vi "Movement Test (Remote Control).vi"() -> ()   [LabVIEW 2019]
uses:
  SubVIs/Move Type.ctl
  LINX-PCA9865 PWM/LINX-PCA9865 PWM.lvclass
  LINX-PCA9865 PWM/LINX-PCA9865 PWM.lvclass/LINX-PCA9865 PWM.ctl
  LINX-PCA9865 PWM/Write LINX Resource.vi
  LINX-PCA9865 PWM/Write I2C Slave Address (0x40).vi
  LINX-PCA9865 PWM/Write LINX I2C Channel.vi
  LINX-PCA9865 PWM/Read LINX Resource.vi
  <vilib>/MakerHub/LINX/Public/Utilities/Open Local.vi
  <vilib>/MediaMongrels Ltd/Message Queue Helper/MessageQueueHelper.lvlib
  <vilib>/MakerHub/LINX/LMH-LINX.lvlib
panel:
  in  "Array":T1[](array[typedef])=[{"Option"="Forward", "Left"=27.0, "Right"=10.0, "Duration"=3.0}, {"Option"="Back", "Left"=-14.0, "Right"=-28.0, "Duration"=3.0}, {"Option"="Left", "Left"=-10.0, "Right"=6.0, "Duration"=0.5}, {"Option"="Right", "Left"=25.0, "Right"=-25.0, "Duration"=0.5}]
  in  "Exit":bool
  in  "Stop":bool
  in  "Left":bool
  in  "Right":bool
  in  "Back":bool
  in  "Forward":bool
  out "Frequency (Hz)":dbl
  out "Drives Enabled?":bool
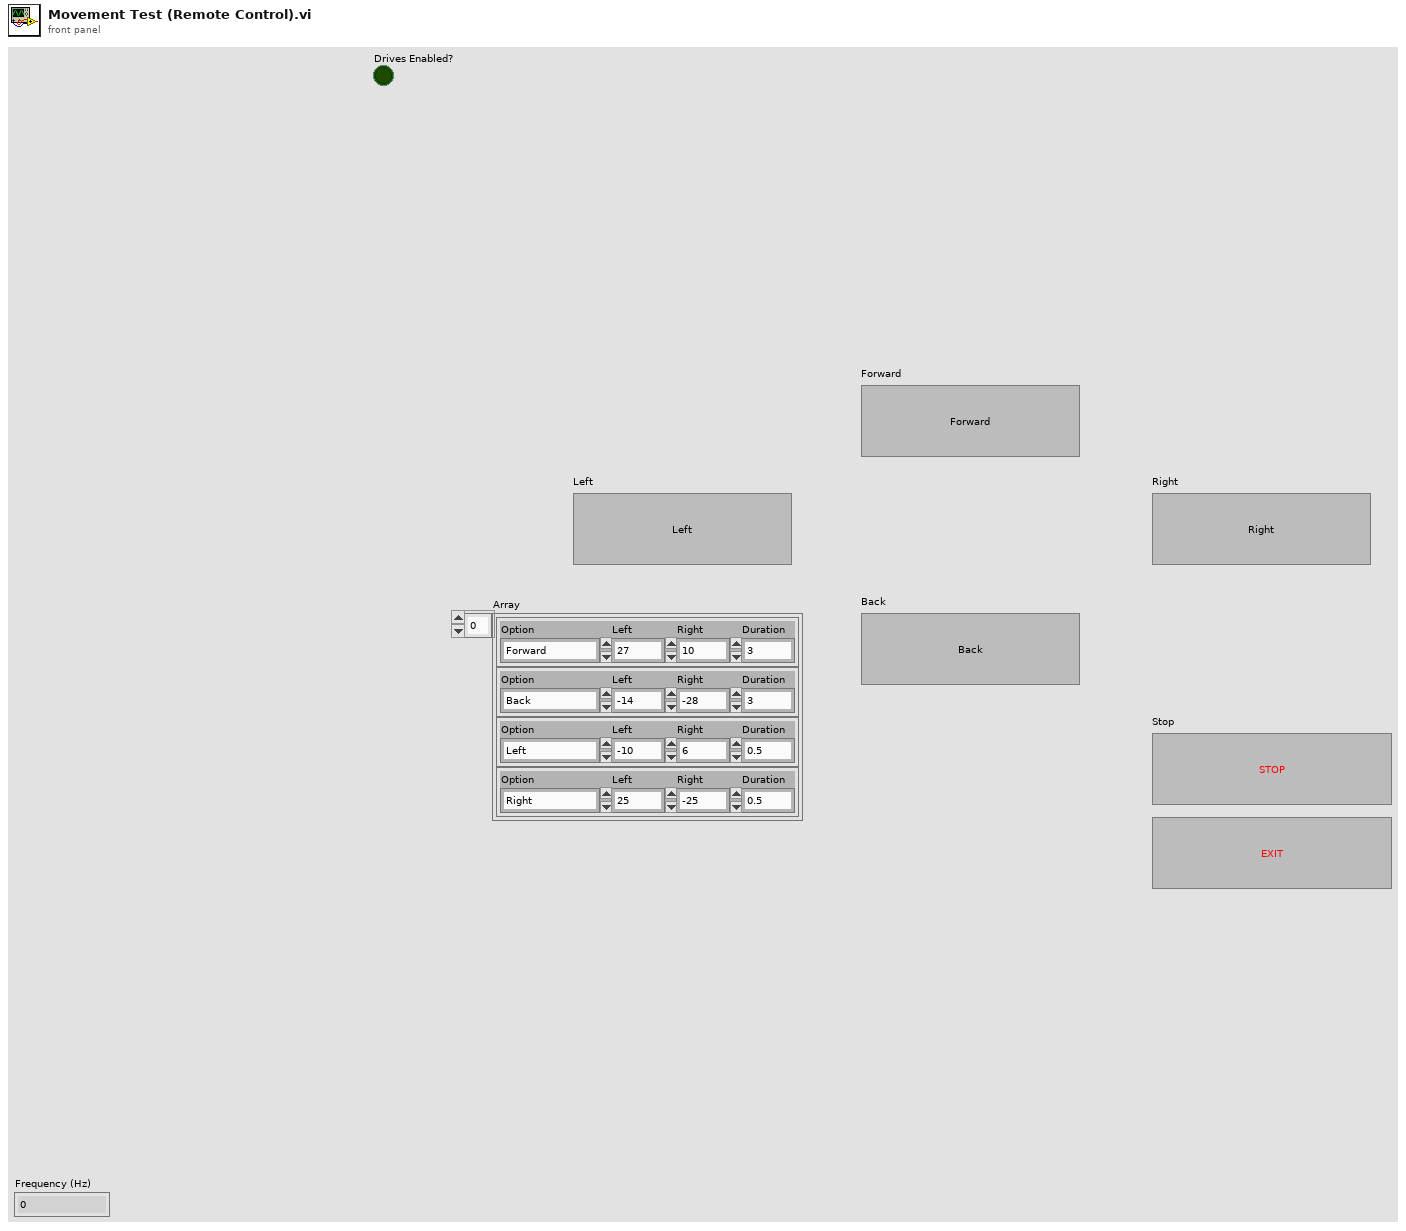
[diagram p1: front panel]
types:
  T1 = typedef "Move Type.ctl" = cluster{"Option":string, "Left":dbl, "Right":dbl, "Duration":dbl}
  T2 = typedef "LMH-LINX.lvlib/LINX Ref.ctl" = cluster{"IO":T3, "Interface":T4, "LINX Device Config":T5}
  T3 = typedef "LMH-LINX.lvlib/Platform.ctl" = enum16{"Remote", "Local"}
  T4 = typedef "LMH-LINX.lvlib/Interface.ctl" = enum16{"Serial", "TCP"}
  T5 = typedef "LMH-LINX.lvlib/Device.lvlib/LINX Device Config.ctl" = cluster{"Interface":T4, "COM Port":refnum<visa-resource-name>, "TCP Configuration":T6, "Device Family":u8, "Device ID":u8, "Device Name":string, "TCP Ref":refnum<k5>, "Channels":T7}
  T6 = typedef "LMH-LINX.lvlib/Device.lvlib/TCP Config.ctl" = cluster{"IP Address":string, "Port":u16}
  T7 = typedef "LMH-LINX.lvlib/Channels.ctl" = cluster{"DI":u8[], "DO":u8[], "AI":u8[], "AO":u8[], "PWM":u8[], "QE":u8[], "UART":u8[], "I2C 2":u8[], "SPI":u8[], "CAN":u8[], "Servo":u8[], "AI Ref (V)":dbl, "AI Resolution (Bits)":u8, "AO Ref (V)":dbl, "AO Resolution (Bits)":u8}
  T8 = enum16{"LED/PWM00", "LED/PWM01", "LED/PWM02", "LED/PWM03", "LED/PWM04", "LED/PWM05", "LED/PWM06", "LED/PWM07", "LED/PWM08", "LED/PWM09", "LED/PWM10", "LED/PWM11", "LED/PWM12", "LED/PWM13", "LED/PWM14", "LED/PWM15"}[]
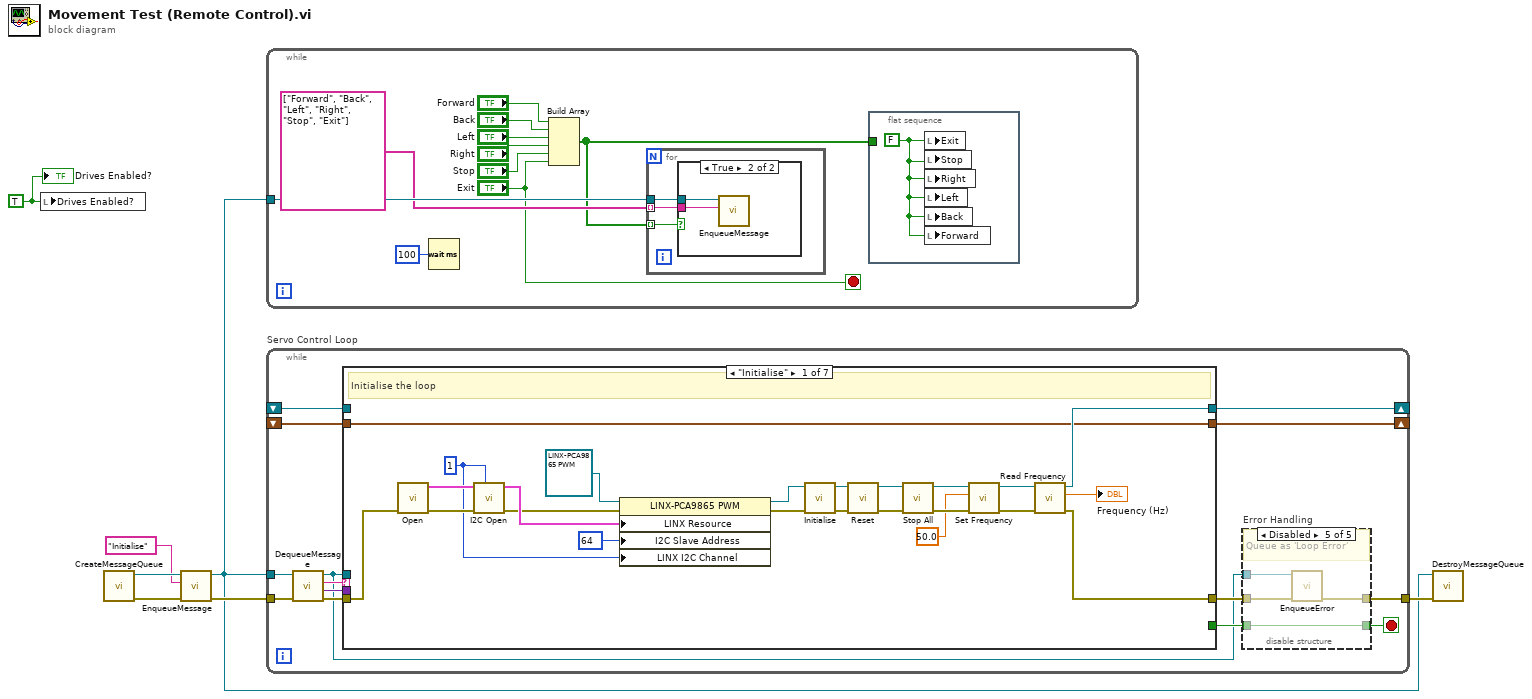
[diagram p0: block diagram]
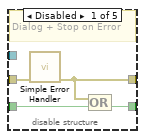
[diagram p3: hidden frame]
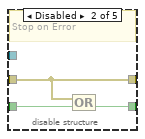
[diagram p4: hidden frame]
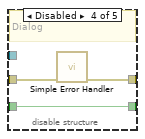
[diagram p6: hidden frame]
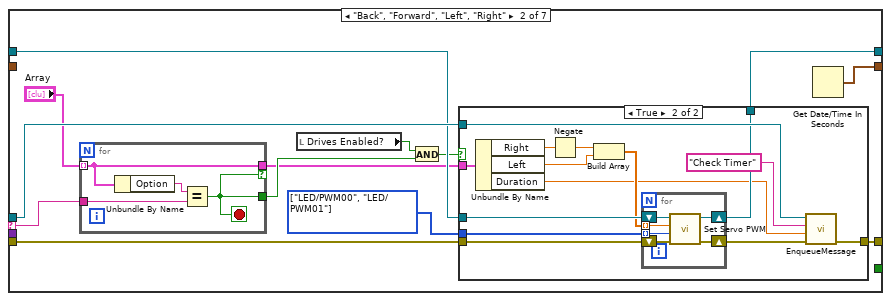
[diagram p7: hidden frame]
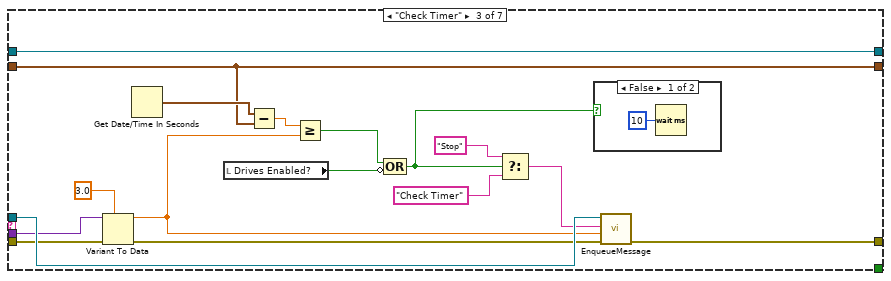
[diagram p9: hidden frame]
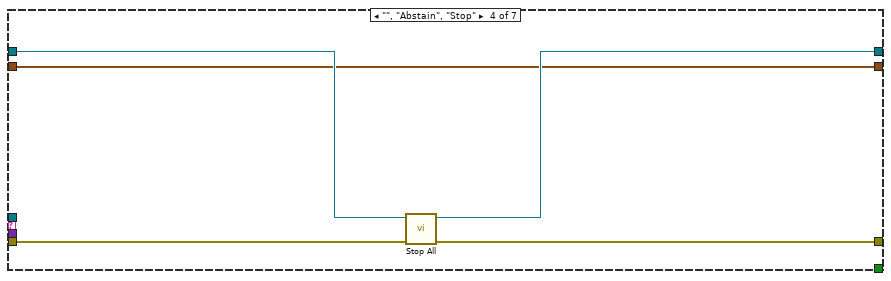
[diagram p11: hidden frame]
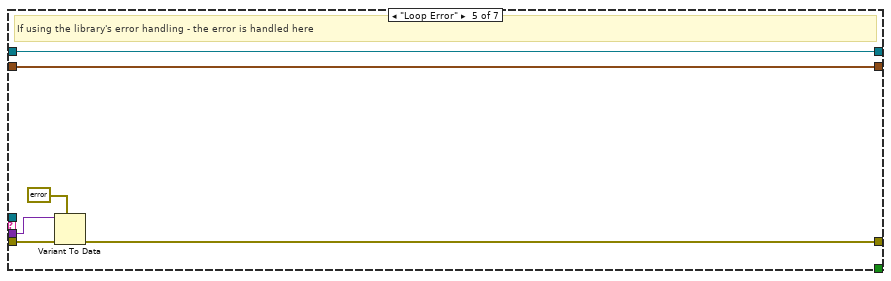
[diagram p12: hidden frame]
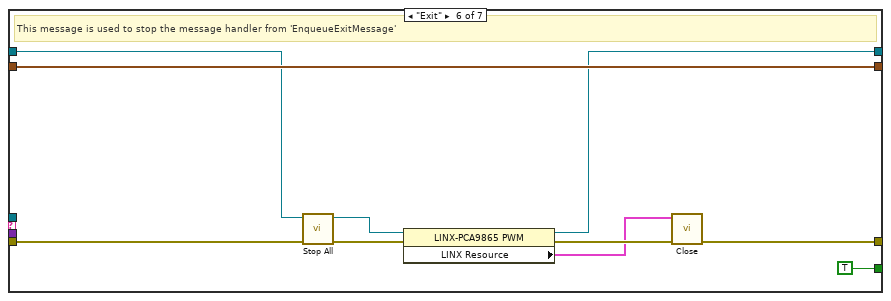
[diagram p13: hidden frame]
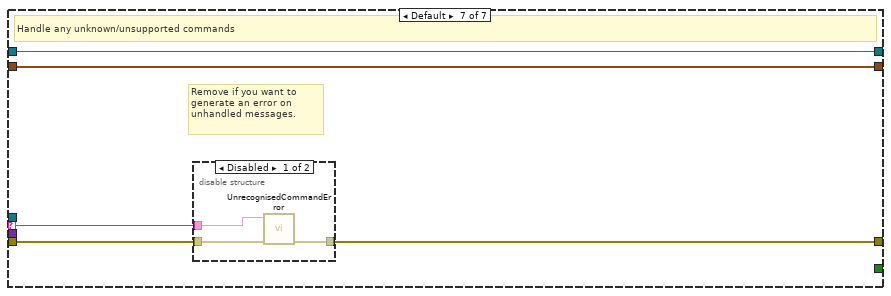
[diagram p14: hidden frame]
diagram:
  w1 = TRUE ("Drives Enabled?")
  n1 = local write "Drives Enabled?"(w1) -> ()
  n2 = call <vilib>:"CreateMessageQueue.vi"() -> ("error out"=w3:errorcluster, "queue out"=w5:refnum<queue>)  [unwired: 9 in, 1 out]
  n3 = call <vilib>:"EnqueueMessage.vi"("error in (no error)"=w3, "Command"="Initialise", "Message Queue in"=w5) -> ("error out"=w6:errorcluster, "Message Queue out"=w2:refnum<queue>)  [unwired: 6 in, 1 out]
  n4 = while {
    tunnel: w2 -> [w17]
    stop <- "Exit" stop-if-true
    n5 = Wait (ms)(milliseconds to wait=u32 100) -> ()  [unwired: 1 out]
    n6 = Build Array("Forward", "Back", "Left", "Right", "Stop", "Exit") -> (w8:bool[])
    n7 = for {
      tunnel: w17 -> [w21]
      tunnel: w8 -> [w20] mode=indexing
      tunnel: string[] ["Forward", "Back", "Left", "Right", "Stop", "Exit"] -> [w19] mode=indexing
      n8 = case shown="True" w20 {
        tunnel: w21 -> [_ w23]
        tunnel: w19 -> [_ w22]
        frame False {
        }
        frame True {
          n9 = call <vilib>:"EnqueueMessage.vi"("Command"=w22, "Message Queue in"=w23) -> ()  [unwired: 7 in, 3 out]
        }
      }
    }
    n10 = flat-sequence {
      tunnel: w8 -> [_]
      frame #0 {
        w18 = FALSE ("Exit")
        n11 = local write "Exit"(w18) -> ()
        n12 = local write "Stop"(w18) -> ()
        n13 = local write "Right"(w18) -> ()
        n14 = local write "Left"(w18) -> ()
        n15 = local write "Back"(w18) -> ()
        n16 = local write "Forward"(w18) -> ()
      }
    }
  }
  n17 = while "Servo Control Loop" {
    tunnel: w6 -> [w37]
    tunnel: w2 -> [w36]
    tunnel: [w29] -> w7
    shift-right: [w27] -> _
    shift-left: _ -> [w26]
    shift-right: [w25] -> _
    shift-left: _ -> [w24]
    stop <- w31 stop-if-true
    n18 = call <vilib>:"DequeueMessage.vi"("error in (no error)"=w37, "Message Queue in"=w36) -> ("error out"=w33:errorcluster, "Data"=w34:variant, "Command"=w35:string, "Message Queue out"=w28:refnum<queue>)  [unwired: 5 in, 1 out]
    n19 = case shown="\"Initialise\"" w35 {
      selector: w35 -> [_ w82 _ _ _ _ w157]
      tunnel: w34 -> [_ _ w118 _ w142 _ _]
      tunnel: w33 -> [w56 w85 w125 w138 w144 w152 w159]
      tunnel: w28 -> [_ w87 w126 _ _ _ _]
      tunnel: [w55 w88 w124 w137 w143 w146 w158] -> w32
      tunnel: [_ _ _ _ _ TRUE _] -> w30
      tunnel: [w57 w83 w132 w135 w140 w149 w156] -> w27
      tunnel: w26 -> [_ w84 w132 w136 w140 w151 w156]
      tunnel: [w54 w89 w130 w134 w139 w153 w155] -> w25
      tunnel: w24 -> [w54 _ w130 w134 w139 w153 w155]
      frame "Initialise" {
        w60 = u8 1 ("I2C Channel")
        # "Initialise the loop"
        n20 = call-poly <vilib>:"Open.vi"("Error In"=w56) -> ("Error Out"=w63:errorcluster, "LINX Resource"=w62:T2)  [unwired: 8 in, 1 out]
        n21 = call <vilib>:"I2C Open.vi"("I2C Channel (0)"=w60, "Error In"=w63, "LINX Resource"=w62) -> ("Error Out"=w64:errorcluster, "LINX Resource"=w65:T2)  [unwired: 7 in]
        n22 = property class="LINX-PCA9865 PWM"(reference=refnum<class "LINX-PCA9865 PWM.lvclass"> refnum ("LINX-PCA9865 PWM.lvclass"), error in=w64, "LINX Resource"=w65, "I2C Slave Address"=u8 64 ("I2C Slave Address (0)"), "LINX I2C Channel"=w60) -> (reference out=w67:refnum<class "LINX-PCA9865 PWM.lvclass">, error out=w66:errorcluster)
        n23 = call-dynamic "Initialise.vi"("error in (no error)"=w66, "PWM in"=w67) -> ("error out"=w70:errorcluster, "PWM out"=w69:refnum<class "LINX-PCA9865 PWM.lvclass">)  [unwired: 8 in]
        n24 = call-dynamic "Reset.vi"("error in (no error)"=w70, "PWM in"=w69) -> ("error out"=w71:errorcluster, "PWM out"=w72:refnum<class "LINX-PCA9865 PWM.lvclass">)  [unwired: 8 in]
        n25 = call-dynamic "Stop All.vi"("error in (no error)"=w71, "LINX-PCA9865 PWM in"=w72) -> ("error out"=w75:errorcluster, "LINX-PCA9865 PWM out"=w76:refnum<class "LINX-PCA9865 PWM.lvclass">)  [unwired: 8 in]
        n26 = call-dynamic "Set Frequency.vi"("error in (no error)"=w75, "Frequency (1000Hz)"=50.0, "PWM in"=w76) -> ("error out"=w73:errorcluster, "PWM out"=w74:refnum<class "LINX-PCA9865 PWM.lvclass">)  [unwired: 7 in]
        n27 = call-dynamic "Read Frequency.vi"("error in (no error)"=w73, "PWM in"=w74) -> ("error out"=w55:errorcluster, "Frequency (Hz)"=→"Frequency (Hz)":dbl, "PWM out"=w57:refnum<class "LINX-PCA9865 PWM.lvclass">)  [unwired: 7 in]
      }
      frame "Back", "Forward", "Left", "Right" {
        w86 = T8 [enum."LED/PWM00", enum."LED/PWM01"] items=["LED/PWM00", "LED/PWM01", "LED/PWM02", "LED/PWM03", "LED/PWM04", "LED/PWM05", "LED/PWM06", "LED/PWM07", "LED/PWM08", "LED/PWM09", "LED/PWM10", "LED/PWM11", "LED/PWM12", "LED/PWM13", "LED/PWM14", "LED/PWM15"] ("LEDn (PWM channel)")
        n28 = for {
          tunnel: "Array" -> [w92] mode=indexing
          tunnel: [w92] -> w78 if=w90
          tunnel: w82 -> [w91]
          tunnel: [w90] -> w79
          stop <- w90 stop-if-true
          n29 = Unbundle By Name(w92) -> ("Option"=w93:string)
          n30 = Equal?(x=w93, y=w91) -> (x = y?=w90:bool)
        }
        n31 = local read "Drives Enabled?"() -> (w81:bool)
        n32 = And(x=w81, y=w79) -> (x .and. y?=w80:bool)
        n33 = case shown="True" w80 {
          tunnel: [w94 w109] -> w88
          tunnel: w87 -> [_ w108]
          tunnel: w86 -> [_ w106]
          tunnel: w85 -> [w94 w105]
          tunnel: w84 -> [w95 w103]
          tunnel: [w95 w102] -> w83
          tunnel: w78 -> [_ w101]
          frame False {
          }
          frame True {
            n34 = Unbundle By Name(w101) -> ("Right"=w100:dbl, "Left"=w99:dbl, "Duration"=w97:dbl)
            n35 = Negate(x=w100) -> (-x=w96:dbl)
            n36 = Build Array(w96, w99) -> (w98:dbl[])
            n37 = for {
              tunnel: w98 -> [w112] mode=indexing
              tunnel: w106 -> [w111] mode=indexing
              shift-right: [w113] -> w102
              shift-left: w103 -> [w115]
              shift-right: [w114] -> w104
              shift-left: w105 -> [w110]
              n38 = call "Set Servo PWM.vi"("error in (no error)"=w110, "LEDn (PWM channel)"=w111, "Servo Speed (-100 to 100%)"=w112, "LINX-PCA9865 PWM in"=w115) -> ("error out"=w114:errorcluster, "LINX-PCA9865 PWM out"=w113:refnum<class "LINX-PCA9865 PWM.lvclass">)  [unwired: 6 in]
            }
            n39 = call <vilib>:"EnqueueMessage.vi"("error in (no error)"=w104, "Data"=w97, "Command"="Check Timer", "Message Queue in"=w108) -> ("error out"=w109:errorcluster)  [unwired: 5 in, 2 out]
          }
        }
        n40 = Get Date/Time In Seconds() -> (seconds since 1Jan1904=w89:timestamp)
      }
      frame "Check Timer" {
        n41 = Variant To Data(error in=w125, type=3.0, Variant=w118) -> (data=w117:dbl, error out=w119:errorcluster)
        n42 = Get Date/Time In Seconds() -> (seconds since 1Jan1904=w131:timestamp)
        n43 = local read "Drives Enabled?"() -> (w127:bool)
        n44 = Subtract(x=w131, y=w130) -> (x-y=w129:dbl)
        n45 = Greater Or Equal?(x=w129, y=w117) -> (x >= y?=w128:bool)
        n46 = Compound Arithmetic op=OR(w128, invert w127) -> (w120:bool)
        n47 = Select(t="Stop", s=w120, f="Check Timer") -> (s? t:f=w121:string)
        n48 = case shown="False" w120 {
          frame False {
            n49 = Wait (ms)(milliseconds to wait=u32 10) -> ()  [unwired: 1 out]
          }
          frame True {
          }
        }
        n50 = call <vilib>:"EnqueueMessage.vi"("error in (no error)"=w119, "Data"=w117, "Command"=w121, "Message Queue in"=w126) -> ("error out"=w124:errorcluster)  [unwired: 5 in, 2 out]
      }
      frame "", "Abstain", "Stop" {
        n51 = call-dynamic "Stop All.vi"("error in (no error)"=w138, "LINX-PCA9865 PWM in"=w136) -> ("error out"=w137:errorcluster, "LINX-PCA9865 PWM out"=w135:refnum<class "LINX-PCA9865 PWM.lvclass">)  [unwired: 8 in]
      }
      frame "Loop Error" {
        # "If using the library's error handling - the error is handled here"
        n52 = Variant To Data(error in=w144, type=errorcluster {"status"=FALSE, "code"=0, "source"=""} ("error constant"), Variant=w142) -> (error out=w143:errorcluster)  [unwired: 1 out]
      }
      frame "Exit" {
        # "This message is used to stop the message handler from 'EnqueueExitMessage'"
        n53 = call-dynamic "Stop All.vi"("error in (no error)"=w152, "LINX-PCA9865 PWM in"=w151) -> ("error out"=w148:errorcluster, "LINX-PCA9865 PWM out"=w150:refnum<class "LINX-PCA9865 PWM.lvclass">)  [unwired: 8 in]
        n54 = property class="LINX-PCA9865 PWM"(reference=w150, error in=w148) -> (reference out=w149:refnum<class "LINX-PCA9865 PWM.lvclass">, error out=w147:errorcluster, "LINX Resource"=w145:T2)
        n55 = call <vilib>:"Close.vi"("Error In"=w147, "LINX Resource"=w145) -> ("Error Out"=w146:errorcluster)  [unwired: 9 in]
      }
      frame Default {
        # "Remove if you want to generate an error on unhandled messages."
        # "Handle any unknown/unsupported commands"
        n56 = disable-structure shown="Disabled" {
          disable-tunnel: w159 -> [w161 w163]
          disable-tunnel: [w162 w163] -> w158
          disable-tunnel: w157 -> [w160 _]
          frame Disabled {
            n57 = call <vilib>:"UnrecognisedCommandError.vi"("error in (no error)"=w161, "Command"=w160) -> ("error out"=w162:errorcluster)  [unwired: 9 in]
          }
          frame Enabled {
          }
        }
      }
    }
    n58 = disable-structure "Error Handling" shown="Disabled" {
      disable-tunnel: w30 -> [w41 w44 w45 w48 w51]
      disable-tunnel: w32 -> [w40 w42 w46 w49 w53]
      disable-tunnel: [w39 w43 w45 w48 w51] -> w31
      disable-tunnel: [w38 w42 w46 w47 w52] -> w29
      disable-tunnel: w28 -> [_ _ _ _ w50]
      frame Disabled {
        # "Dialog + Stop on Error"
        n59 = call <vilib>:"Simple Error Handler.vi"("error in (no error)"=w40) -> ("error out"=w38:errorcluster)  [unwired: 4 in, 4 out]
        n60 = Compound Arithmetic op=OR(w38, w41) -> (w39:bool)
      }
      frame Disabled {
        # "Stop on Error"
        n61 = Compound Arithmetic op=OR(w42, w44) -> (w43:bool)
      }
      frame Enabled {
        # "Continue on Error"
      }
      frame Disabled {
        # "Dialog"
        n62 = call <vilib>:"Simple Error Handler.vi"("error in (no error)"=w49) -> ("error out"=w47:errorcluster)  [unwired: 4 in, 4 out]
      }
      frame Disabled {
        # "Queue as 'Loop Error'"
        n63 = call <vilib>:"EnqueueError.vi"("error in (no error)"=w53, "Message Queue in"=w50) -> ("error out"=w52:errorcluster)  [unwired: 9 in]
      }
    }
  }
  n64 = call <vilib>:"DestroyMessageQueue.vi"("error in (no error)"=w7, "Message Queue in"=w2) -> ()  [unwired: 9 in, 1 out]
  "Drives Enabled?" <- w1
